vi "Laser_COM.vi"() -> ()   [LabVIEW 2014]
uses:
  <vilib>/Instr/_visa.llb/Select Event Type.ctl
  <vilib>/Instr/_visa.llb/VISA Configure Serial Port (Instr).vi
panel:
  out "on/off? 5":bool
  in  "Laser":bool caption="Основной Лазер"
  out "on/off? 4":bool caption="Излучение включено!"
  out "on/off? 3":bool
  out "on/off? 2":bool
  out "head temp":dbl caption="Темп. излучателя" format="%#_g °C"
  in  "Send":bool
  in  "write buffer":string caption="Передать команду"
  out "LaserOn":bool
  in  "term_char":i16=13 format="%x"
  in  "SwitchLaser":bool
  out "SN:":string
  out "Лазер: ID:":string
  out "on/off?":bool
  out "module temp":dbl caption="Темп. модуля" format="%#_g °C"
  in  "Power":dbl(slide)=10.0 caption="Мощность излучения, %" min=10.0 max=100.0 step=0.5 scale=0.0..100.0 scale format="%#.2g"
  in  "Laser pilot":bool caption="Лазер пилот"
  in  "COM":refnum<visa-resource-name>="COM1" caption="Laser COM-port"
  out "read buffer":string caption="ОТВЕТ:"
  out "error out":errorcluster
  in  "error in (no error)":errorcluster
  # "termination char\n(0xD = CR)"
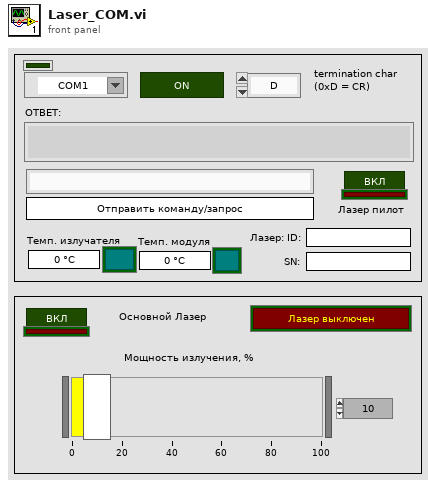
[diagram p1: front panel]
types:
  T1 = typedef "Select Event Type.ctl" = u32
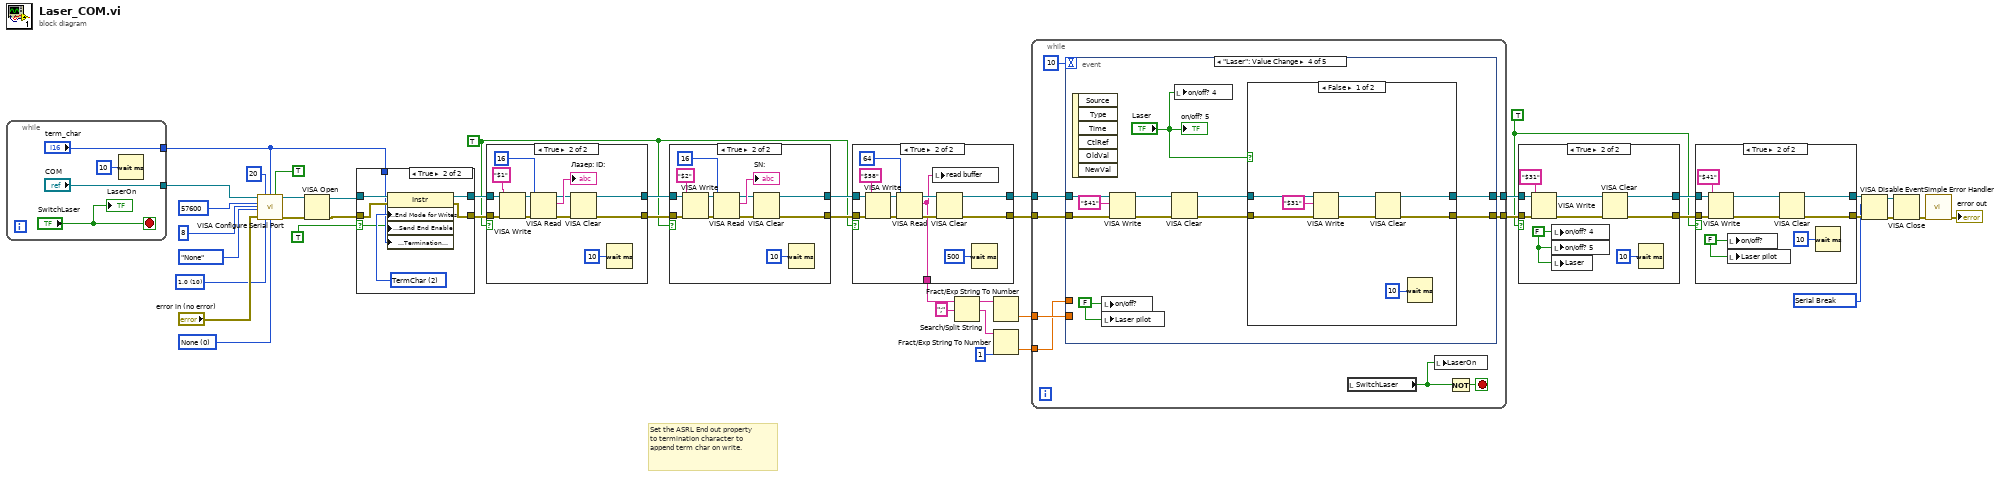
[diagram p0: block diagram]
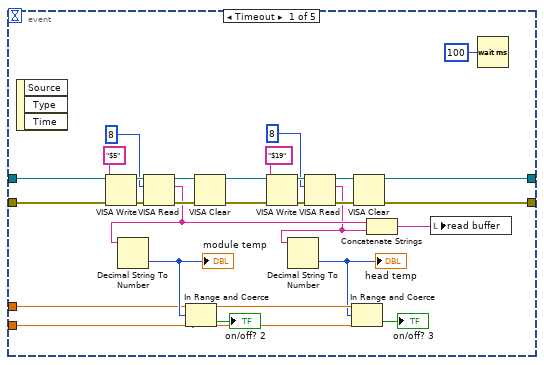
[diagram p7: hidden frame]
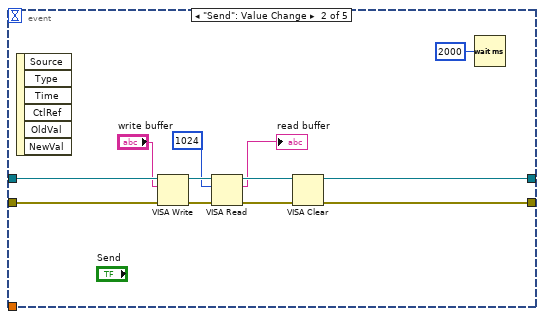
[diagram p8: hidden frame]
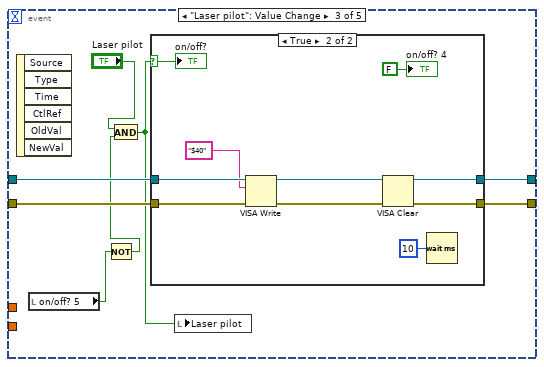
[diagram p9: hidden frame]
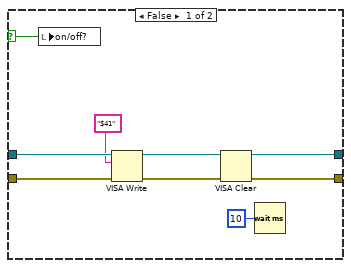
[diagram p10: hidden frame]
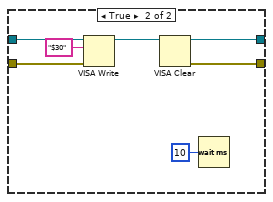
[diagram p11: hidden frame]
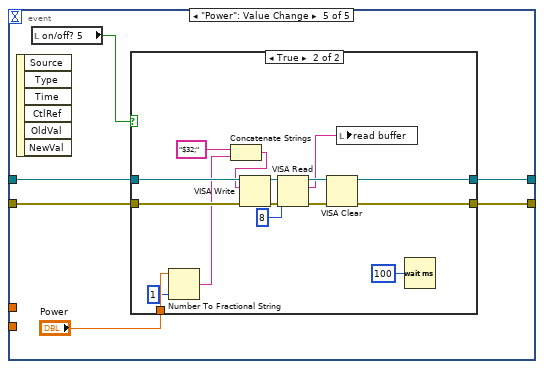
[diagram p12: hidden frame]
diagram:
  w1 = T1 1073684515 items=["Service Request"=1073684491, "Trigger"=3221168138, "Clear"=1073684493, "VXI Signal"=1073684512, "VXI/VME Interrupt"=3221168161, "VXI/VME Sysfail"=1073684509, "VXI/VME Sysreset"=1073684510, "GPIB CIC"=1073684498, "GPIB Talk"=1073684499, "GPIB Listen"=1073684500, "PXI Interrupt"=1073684514, "Serial Break"=1073684515, "Serial TermChar"=1073684516, "Serial CTS"=1073684521, "Serial DSR"=1073684522, "Serial DCD"=1073684524, "Serial RI"=1073684526, "Serial Character"=1073684533, "USB Interrupt"=1073684535, "All Enabled"=1073709055] ("Event Type")
  w6 = TRUE
  w25 = u16 0 items=["None", "XON/XOFF", "RTS/CTS", "XON/XOFF & RTS/CTS", "DTR/DSR", "XON/XOFF & DTR/DSR"] ("flow control (0:none)")
  w17 = TRUE
  w36 = u16 10 items=["1.0"=10, "1.5"=15, "2.0"=20] ("stop bits (10: 1 bit)")
  # "Set the ASRL End out property to termination character to append term char on write."
  n1 = while {
    tunnel: ["COM"] -> w24
    tunnel: ["term_char"] -> w23
    stop <- "SwitchLaser" stop-if-true
    n2 = Wait (ms)(milliseconds to wait=u32 10) -> ()  [unwired: 1 out]
    "LaserOn" <- "SwitchLaser"
  }
  n3 = call-poly "VISA Configure Serial Port"("VISA resource name"=w24, "timeout (10sec)"=u32 20, "termination char\n(0xA = '\\n' = LF)"=w23, "Enable Termination\nChar (T)"=TRUE ("Enable Termination\nChar (T)"), "baud rate (9600)"=u32 57600 ("baud rate"), "data bits (8)"=u16 8, "parity (0:none)"=enum16{"None", "Odd", "Even", "Mark", "Space"}."None", "error in (no error)"="error in (no error)", "stop bits (10: 1 bit)"=w36, "flow control (0:none)"=w25) -> ("VISA resource name out"=w39:refnum<visa-resource-name>, "error out"=w38:errorcluster)  [unwired: 4 in]
  n4 = VISA Open(error in (no error)=w38, VISA resource name=w39) -> (VISA resource name=w33:refnum<visa-resource-name>, error out=w34:errorcluster)  [unwired: 3 in]
  n5 = case shown="True" TRUE ("End write with termination character?") {
    selector: TRUE ("End write with termination character?") -> [_ w50]
    tunnel: w33 -> [w48 w56]
    tunnel: w34 -> [w49 w55]
    tunnel: [w48 w54] -> w29
    tunnel: [w49 w53] -> w28
    tunnel: w23 -> [_ w51]
    frame False {
    }
    frame True {
      w52 = u16 2 items=["None", "LastBit", "TermChar", "Break"] ("Serial Settings:Serial End Mode for Writes")
      n6 = property class="Instr"(reference=w56, error in=w55, "Serial Settings:End Mode for Writes"=w52, "Message Based Settings:Send End Enable"=w50, "Message Based Settings:Termination Character"=w51) -> (reference out=w54:refnum<visa-resource-name>, error out=w53:errorcluster)
    }
  }
  n7 = case shown="True" w17 {
    tunnel: w29 -> [w58 w68]
    tunnel: w28 -> [w57 w67]
    tunnel: [w58 w62] -> w27
    tunnel: [w57 w61] -> w26
    frame False {
    }
    frame True {
      n8 = VISA Write(VISA resource name=w68, write buffer="$1", error in (no error)=w67) -> (VISA resource name out=w69:refnum<visa-resource-name>, error out=w70:errorcluster)  [unwired: 1 out]
      n9 = VISA Read(VISA resource name=w69, byte count=u32 16, error in (no error)=w70) -> (VISA resource name out=w64:refnum<visa-resource-name>, read buffer=→"Лазер: ID:":string, error out=w63:errorcluster)  [unwired: 1 out]
      n10 = VISA Clear(VISA resource name=w64, error in (no error)=w63) -> (VISA resource name out=w62:refnum<visa-resource-name>, error out=w61:errorcluster)
      n11 = Wait (ms)(milliseconds to wait=u32 10) -> ()  [unwired: 1 out]
    }
  }
  n12 = case shown="True" w17 {
    tunnel: w27 -> [w72 w82]
    tunnel: w26 -> [w71 w81]
    tunnel: [w72 w76] -> w20
    tunnel: [w71 w75] -> w19
    frame False {
    }
    frame True {
      n13 = VISA Write(VISA resource name=w82, write buffer="$2", error in (no error)=w81) -> (VISA resource name out=w83:refnum<visa-resource-name>, error out=w84:errorcluster)  [unwired: 1 out]
      n14 = VISA Read(VISA resource name=w83, byte count=u32 16, error in (no error)=w84) -> (VISA resource name out=w78:refnum<visa-resource-name>, read buffer=→"SN:":string, error out=w77:errorcluster)  [unwired: 1 out]
      n15 = VISA Clear(VISA resource name=w78, error in (no error)=w77) -> (VISA resource name out=w76:refnum<visa-resource-name>, error out=w75:errorcluster)
      n16 = Wait (ms)(milliseconds to wait=u32 10) -> ()  [unwired: 1 out]
    }
  }
  n17 = case shown="True" w17 {
    tunnel: w20 -> [w86 w96]
    tunnel: w19 -> [w85 w95]
    tunnel: [w86 w91] -> w22
    tunnel: [w85 w90] -> w21
    tunnel: [_ w88] -> w13
    frame False {
    }
    frame True {
      n18 = VISA Write(VISA resource name=w96, write buffer="$58", error in (no error)=w95) -> (VISA resource name out=w97:refnum<visa-resource-name>, error out=w98:errorcluster)  [unwired: 1 out]
      n19 = VISA Read(VISA resource name=w97, byte count=u32 64, error in (no error)=w98) -> (VISA resource name out=w93:refnum<visa-resource-name>, read buffer=w88:string, error out=w92:errorcluster)  [unwired: 1 out]
      n20 = local write "read buffer"(w88) -> ()
      n21 = VISA Clear(VISA resource name=w93, error in (no error)=w92) -> (VISA resource name out=w91:refnum<visa-resource-name>, error out=w90:errorcluster)
      n22 = Wait (ms)(milliseconds to wait=u32 500) -> ()  [unwired: 1 out]
    }
  }
  n23 = Search/Split String(string=w13, search string/char (-)=";") -> (substring before match=w16:string, match + rest of string=w15:string)  [unwired: 1 in, 1 out]
  n24 = Fract/Exp String To Number(string=w16) -> (number=w12:dbl)  [unwired: 3 in, 1 out]
  n25 = Fract/Exp String To Number(string=w15, offset=1) -> (number=w11:dbl)  [unwired: 2 in, 1 out]
  n26 = while {
    tunnel: w21 -> [w102]
    tunnel: w22 -> [w103]
    tunnel: [w105] -> w10
    tunnel: [w104] -> w9
    tunnel: w12 -> [w100]
    tunnel: w11 -> [w99]
    stop <- w107 stop-if-true
    n27 = event shown="[3] \"Laser\": Value Change" {
      selector: _ -> [_ _ _ _ _]
      dyn-events: _ -> [_ _ _ _ _]
      timeout: 10 -> [_ _ _ _ _]
      tunnel: w103 -> [w129 w147 w155 w184 w205]
      tunnel: w102 -> [w130 w146 w154 w183 w204]
      tunnel: [w123 w141 w153 w179 w203] -> w105
      tunnel: [w122 w140 w152 w178 w202] -> w104
      tunnel: w100 -> [w111 _ _ _ _]
      tunnel: w99 -> [w112 _ _ _ _]
      event Timeout {
        n28 = event-data() -> ()  [unwired: 1 in, 3 out]
        n29 = VISA Write(VISA resource name=w129, write buffer="$5", error in (no error)=w130) -> (VISA resource name out=w134:refnum<visa-resource-name>, error out=w135:errorcluster)  [unwired: 1 out]
        n30 = VISA Read(VISA resource name=w134, byte count=u32 8, error in (no error)=w135) -> (VISA resource name out=w132:refnum<visa-resource-name>, read buffer=w118:string, error out=w131:errorcluster)  [unwired: 1 out]
        n31 = Decimal String To Number(string=w118) -> (number=w115:i32)  [unwired: 2 in, 1 out]
        "module temp" <- w115
        n32 = In Range and Coerce(upper limit=w112, x=w115, lower limit=w111) -> (In Range?=→"on/off? 2":bool)  [unwired: 1 out]
        n33 = VISA Clear(VISA resource name=w132, error in (no error)=w131) -> (VISA resource name out=w121:refnum<visa-resource-name>, error out=w120:errorcluster)
        n34 = VISA Write(VISA resource name=w121, write buffer="$19", error in (no error)=w120) -> (VISA resource name out=w127:refnum<visa-resource-name>, error out=w128:errorcluster)  [unwired: 1 out]
        n35 = VISA Read(VISA resource name=w127, byte count=u32 8, error in (no error)=w128) -> (VISA resource name out=w125:refnum<visa-resource-name>, read buffer=w117:string, error out=w124:errorcluster)  [unwired: 1 out]
        n36 = Decimal String To Number(string=w117) -> (number=w110:i32)  [unwired: 2 in, 1 out]
        "head temp" <- w110
        n37 = In Range and Coerce(upper limit=w112, x=w110, lower limit=w111) -> (In Range?=→"on/off? 3":bool)  [unwired: 1 out]
        n38 = VISA Clear(VISA resource name=w125, error in (no error)=w124) -> (VISA resource name out=w123:refnum<visa-resource-name>, error out=w122:errorcluster)
        n39 = Concatenate Strings(w118, w117) -> (w116:string)
        n40 = local write "read buffer"(w116) -> ()
        n41 = Wait (ms)(milliseconds to wait=u32 100) -> ()  [unwired: 1 out]
      }
      event "Send": Value Change {
        n42 = event-data() -> ()  [unwired: 1 in, 6 out]
        n43 = VISA Write(VISA resource name=w147, write buffer="write buffer", error in (no error)=w146) -> (VISA resource name out=w145:refnum<visa-resource-name>, error out=w144:errorcluster)  [unwired: 1 out]
        n44 = VISA Read(VISA resource name=w145, byte count=u32 1024, error in (no error)=w144) -> (VISA resource name out=w143:refnum<visa-resource-name>, read buffer=→"read buffer":string, error out=w142:errorcluster)  [unwired: 1 out]
        n45 = VISA Clear(VISA resource name=w143, error in (no error)=w142) -> (VISA resource name out=w141:refnum<visa-resource-name>, error out=w140:errorcluster)
        n46 = Wait (ms)(milliseconds to wait=u32 2000) -> ()  [unwired: 1 out]
      }
      event "Laser pilot": Value Change {
        n47 = event-data() -> ()  [unwired: 1 in, 6 out]
        n48 = local read "on/off? 5"() -> (w151:bool)
        n49 = Not(x=w151) -> (.not. x?=w149:bool)
        n50 = And(x="Laser pilot", y=w149) -> (x .and. y?=w148:bool)
        n51 = case shown="True" w148 {
          selector: w148 -> [w162 w172]
          tunnel: w155 -> [w164 w174]
          tunnel: w154 -> [w163 w173]
          tunnel: [w159 w169] -> w153
          tunnel: [w158 w168] -> w152
          frame False {
            n52 = local write "on/off?"(w162) -> ()
            n53 = VISA Write(VISA resource name=w164, write buffer="$41", error in (no error)=w163) -> (VISA resource name out=w157:refnum<visa-resource-name>, error out=w156:errorcluster)  [unwired: 1 out]
            n54 = VISA Clear(VISA resource name=w157, error in (no error)=w156) -> (VISA resource name out=w159:refnum<visa-resource-name>, error out=w158:errorcluster)
            n55 = Wait (ms)(milliseconds to wait=u32 10 ("millisecond multiple")) -> ()  [unwired: 1 out]
          }
          frame True {
            n56 = VISA Write(VISA resource name=w174, write buffer="$40", error in (no error)=w173) -> (VISA resource name out=w166:refnum<visa-resource-name>, error out=w165:errorcluster)  [unwired: 1 out]
            n57 = VISA Clear(VISA resource name=w166, error in (no error)=w165) -> (VISA resource name out=w169:refnum<visa-resource-name>, error out=w168:errorcluster)
            n58 = Wait (ms)(milliseconds to wait=u32 10 ("millisecond multiple")) -> ()  [unwired: 1 out]
            "on/off?" <- w172
            "on/off? 4" <- FALSE ("on/off? 4")
          }
        }
        n59 = local write "Laser pilot"(w148) -> ()
      }
      event "Laser": Value Change {
        w177 = FALSE ("on/off?")
        n60 = event-data() -> ()  [unwired: 1 in, 6 out]
        n61 = local write "on/off?"(w177) -> ()
        n62 = local write "Laser pilot"(w177) -> ()
        n63 = VISA Write(VISA resource name=w184, write buffer="$41", error in (no error)=w183) -> (VISA resource name out=w176:refnum<visa-resource-name>, error out=w175:errorcluster)  [unwired: 1 out]
        n64 = VISA Clear(VISA resource name=w176, error in (no error)=w175) -> (VISA resource name out=w181:refnum<visa-resource-name>, error out=w180:errorcluster)
        n65 = local write "on/off? 4"("Laser") -> ()
        n66 = case shown="False" "Laser" {
          tunnel: w181 -> [w192 w199]
          tunnel: w180 -> [w191 w198]
          tunnel: [w190 w197] -> w179
          tunnel: [w189 w196] -> w178
          frame False {
            n67 = VISA Write(VISA resource name=w192, write buffer="$31", error in (no error)=w191) -> (VISA resource name out=w186:refnum<visa-resource-name>, error out=w187:errorcluster)  [unwired: 1 out]
            n68 = VISA Clear(VISA resource name=w186, error in (no error)=w187) -> (VISA resource name out=w190:refnum<visa-resource-name>, error out=w189:errorcluster)
            n69 = Wait (ms)(milliseconds to wait=u32 10) -> ()  [unwired: 1 out]
          }
          frame True {
            n70 = VISA Write(VISA resource name=w199, write buffer="$30", error in (no error)=w198) -> (VISA resource name out=w194:refnum<visa-resource-name>)  [unwired: 2 out]
            n71 = VISA Clear(VISA resource name=w194) -> (VISA resource name out=w197:refnum<visa-resource-name>, error out=w196:errorcluster)  [unwired: 1 in]
            n72 = Wait (ms)(milliseconds to wait=u32 10) -> ()  [unwired: 1 out]
          }
        }
        "on/off? 5" <- "Laser"
      }
      event "Power": Value Change {
        n73 = event-data() -> ()  [unwired: 1 in, 6 out]
        n74 = local read "on/off? 5"() -> (w206:bool)
        n75 = case shown="True" w206 {
          tunnel: w205 -> [w208 w220]
          tunnel: w204 -> [w207 w219]
          tunnel: [w208 w218] -> w203
          tunnel: [w207 w217] -> w202
          tunnel: "Power" -> [_ w214]
          frame False {
          }
          frame True {
            n76 = Number To Fractional String(number=w214, precision (6)=i16 1) -> (F-format string=w213:string)  [unwired: 2 in]
            n77 = Concatenate Strings("$32;" ("write buffer"), w213) -> (w215:string)
            n78 = VISA Write(VISA resource name=w220, write buffer=w215, error in (no error)=w219) -> (VISA resource name out=w222:refnum<visa-resource-name>, error out=w221:errorcluster)  [unwired: 1 out]
            n79 = VISA Read(VISA resource name=w222, byte count=u32 8, error in (no error)=w221) -> (VISA resource name out=w223:refnum<visa-resource-name>, read buffer=w210:string, error out=w224:errorcluster)  [unwired: 1 out]
            n80 = VISA Clear(VISA resource name=w223, error in (no error)=w224) -> (VISA resource name out=w218:refnum<visa-resource-name>, error out=w217:errorcluster)
            n81 = local write "read buffer"(w210) -> ()
            n82 = Wait (ms)(milliseconds to wait=u32 100) -> ()  [unwired: 1 out]
          }
        }
      }
    }
    n83 = local read "SwitchLaser"() -> (w106:bool)
    n84 = local write "LaserOn"(w106) -> ()
    n85 = Not(x=w106) -> (.not. x?=w107:bool)
  }
  n86 = case shown="True" w6 {
    tunnel: w10 -> [w226 w235]
    tunnel: w9 -> [w225 w234]
    tunnel: [w226 w232] -> w8
    tunnel: [w225 w231] -> w7
    frame False {
    }
    frame True {
      w229 = FALSE ("on/off? 4")
      n87 = VISA Write(VISA resource name=w235, write buffer="$31", error in (no error)=w234) -> (VISA resource name out=w228:refnum<visa-resource-name>, error out=w227:errorcluster)  [unwired: 1 out]
      n88 = local write "on/off? 4"(w229) -> ()
      n89 = local write "on/off? 5"(w229) -> ()
      n90 = local write "Laser"(w229) -> ()
      n91 = VISA Clear(VISA resource name=w228, error in (no error)=w227) -> (VISA resource name out=w232:refnum<visa-resource-name>, error out=w231:errorcluster)
      n92 = Wait (ms)(milliseconds to wait=u32 10) -> ()  [unwired: 1 out]
    }
  }
  n93 = case shown="True" w6 {
    tunnel: w8 -> [w237 w246]
    tunnel: w7 -> [w236 w245]
    tunnel: [w237 w243] -> w5
    tunnel: [w236 w242] -> w3
    frame False {
    }
    frame True {
      w240 = FALSE ("on/off?")
      n94 = VISA Write(VISA resource name=w246, write buffer="$41", error in (no error)=w245) -> (VISA resource name out=w239:refnum<visa-resource-name>, error out=w238:errorcluster)  [unwired: 1 out]
      n95 = local write "on/off?"(w240) -> ()
      n96 = local write "Laser pilot"(w240) -> ()
      n97 = VISA Clear(VISA resource name=w239, error in (no error)=w238) -> (VISA resource name out=w243:refnum<visa-resource-name>, error out=w242:errorcluster)
      n98 = Wait (ms)(milliseconds to wait=u32 10) -> ()  [unwired: 1 out]
    }
  }
  n99 = VISA Disable Event(8:w3, 10:w1, 11:w5) -> (0:w2:errorcluster, 3:w4:refnum<visa-resource-name>)  [unwired: 1 out]
  n100 = VISA Close(VISA resource name=w4, error in (no error)=w2) -> (error out=w30:errorcluster)
  n101 = call <vilib>:"Simple Error Handler.vi"("error in (no error)"=w30) -> ("error out"=→"error out":errorcluster)  [unwired: 4 in, 4 out]
